vi "DEMO_positioner.vi"(8 "error in":errorcluster, 10 "command":string, 11 "reference in":refnum<vi>) -> (0 "error out":errorcluster)   [LabVIEW 2010]
panel:
  in  "front panel VI Refnum":refnum<vi>
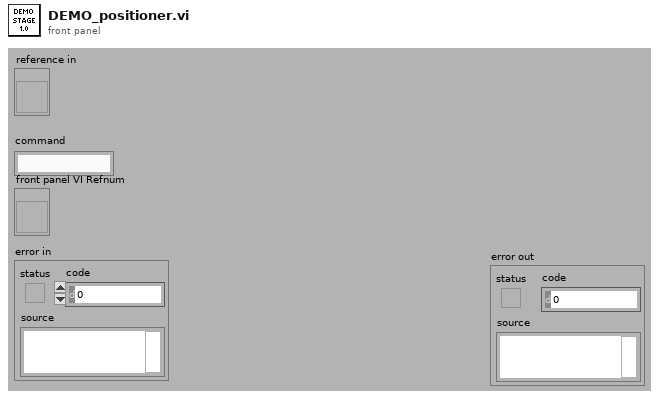
[diagram p1: front panel]
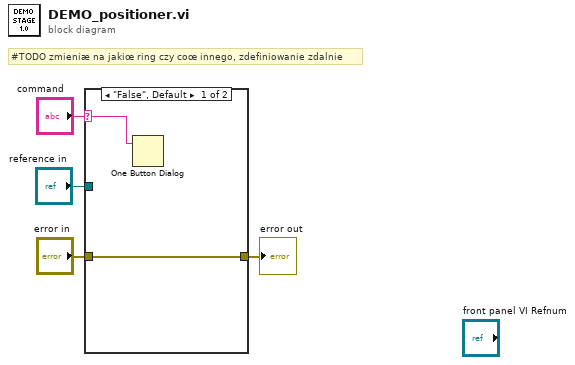
[diagram p0: block diagram]
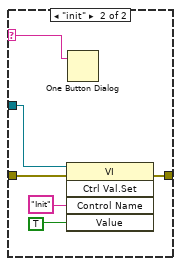
[diagram p2: hidden frame]
diagram:
  # "#TODO zmieniæ na jakiœ ring czy coœ innego, zdefiniowanie zdalnie"
  n1 = case shown="\"False\", Default" "command" {
    selector: "command" -> [w5 w7]
    tunnel: "reference in" -> [_ w12]
    tunnel: "error in" -> [w6 w10]
    tunnel: [w6 w9] -> w2
    frame "False", Default {
      n2 = One Button Dialog(message=w5) -> ()  [unwired: 1 in, 1 out]
    }
    frame "init" {
      n3 = invoke class="VI" method="Ctrl Val.Set"(reference=w12, error in=w10, "Control Name"="Init", "Value"=TRUE) -> (error out=w9:errorcluster)  [unwired: 1 in, 4 out]
      n4 = One Button Dialog(message=w7) -> ()  [unwired: 1 in, 1 out]
    }
  }
  "error out" <- w2
